vi "HashTable Demo.vi"() -> ()   [LabVIEW 2011]
uses:
  HashTable.lvclass
panel:
  out "New Count":i32
  out "Count":i32
  out "New Value":variant caption="Value"
  out "Value":variant
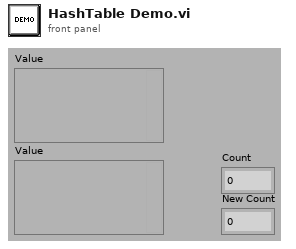
[diagram p1: front panel]
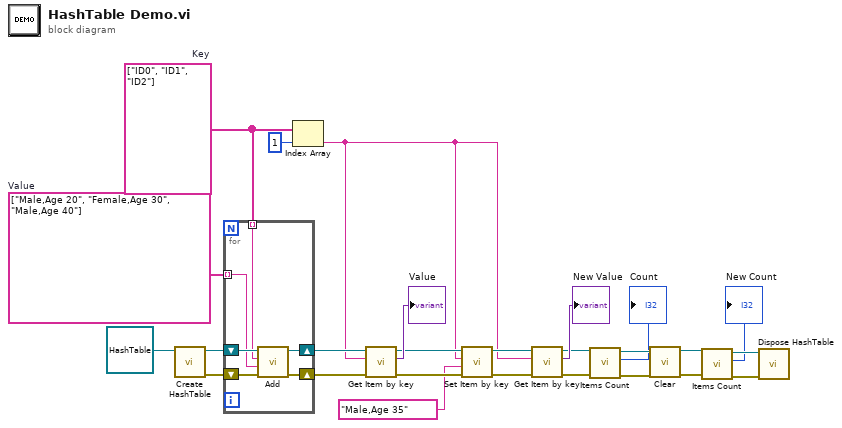
[diagram p0: block diagram]
diagram:
  w23 = string[] ["Male,Age 20", "Female,Age 30", "Male,Age 40"]  # Value
  w20 = string[] ["ID0", "ID1", "ID2"]  # Key
  n1 = call "Create HashTable.vi"("HashTable 输入"=refnum<class "HashTable.lvclass"> refnum ("HashTable.lvclass")) -> ("error out"=w24:errorcluster, "HashTable 输出"=w25:refnum<class "HashTable.lvclass">)  [unwired: 9 in]
  n2 = for {
    tunnel: w20 -> [w28] mode=indexing
    shift-right: [w29] -> w22
    shift-left: w25 -> [w30]
    shift-right: [w31] -> w21
    shift-left: w24 -> [w32]
    tunnel: w23 -> [w27] mode=indexing
    n3 = call "Add.vi"("error in (no error)"=w32, "Value"=w27, "Key"=w28, "HashTable 输入"=w30) -> ("error out"=w31:errorcluster, "HashTable 输出"=w29:refnum<class "HashTable.lvclass">)  [unwired: 6 in]
  }
  n4 = Index Array(array=w20, index=1 ("索引")) -> (element=w12:string)
  n5 = call "Get Item by key.vi"("error in (no error)"=w21, "Key"=w12, "HashTable 输入"=w22) -> ("error out"=w16:errorcluster, "Value"=→"Value":variant, "HashTable 输出"=w17:refnum<class "HashTable.lvclass">)  [unwired: 6 in]
  n6 = call "Set Item by key.vi"("error in (no error)"=w16, "Value"="Male,Age 35", "Key"=w12, "HashTable 输入"=w17) -> ("error out"=w13:errorcluster, "HashTable 输出"=w14:refnum<class "HashTable.lvclass">)  [unwired: 6 in]
  n7 = call "Get Item by key.vi"("error in (no error)"=w13, "Key"=w12, "HashTable 输入"=w14) -> ("error out"=w9:errorcluster, "Value"=→"New Value":variant, "HashTable 输出"=w10:refnum<class "HashTable.lvclass">)  [unwired: 6 in]
  n8 = call "Items Count.vi"("error in (no error)"=w9, "HashTable 输入"=w10) -> ("error out"=w7:errorcluster, "Count"=→"Count":i32, "HashTable 输出"=w8:refnum<class "HashTable.lvclass">)  [unwired: 7 in]
  n9 = call "Clear.vi"("error in (no error)"=w7, "HashTable 输入"=w8) -> ("error out"=w4:errorcluster, "HashTable 输出"=w5:refnum<class "HashTable.lvclass">)  [unwired: 8 in]
  n10 = call "Items Count.vi"("error in (no error)"=w4, "HashTable 输入"=w5) -> ("error out"=w2:errorcluster, "Count"=→"New Count":i32, "HashTable 输出"=w3:refnum<class "HashTable.lvclass">)  [unwired: 7 in]
  n11 = call "Dispose HashTable.vi"("error in (no error)"=w2, "HashTable 输入"=w3) -> ()  [unwired: 8 in, 2 out]
